vi "Am I Beside Destination.vi"(2 "Max Distance per step":cdb, 3 "Destination Location":cdb, 4 "Allowed Directions to move":T1[](array[typedef]), 5 "Current Location":cdb) -> (0 "Am I beside Destination ?":bool, 1 "Direction to Destination":T1)   [LabVIEW 2020, in "AoC 2022.lvlib"]
uses:
  AoC 2022.lvlib
  Direction.ctl
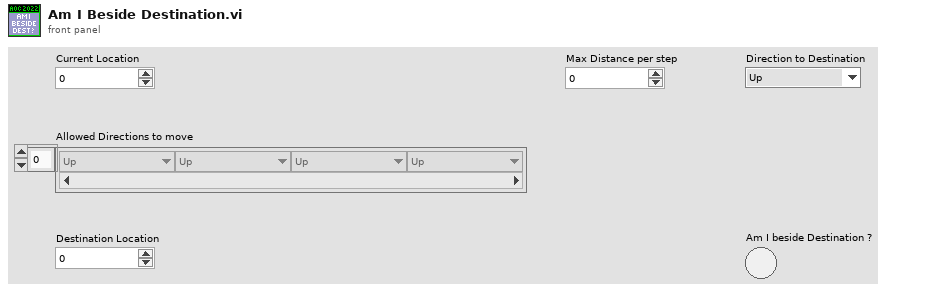
[diagram p1: front panel]
types:
  T1 = typedef "AoC 2022.lvlib/Direction.ctl" = enum16{"Up", "UpRight", "Right", "DownRight", "Down", "DownLeft", "Left", "UpLeft", "Stay"}
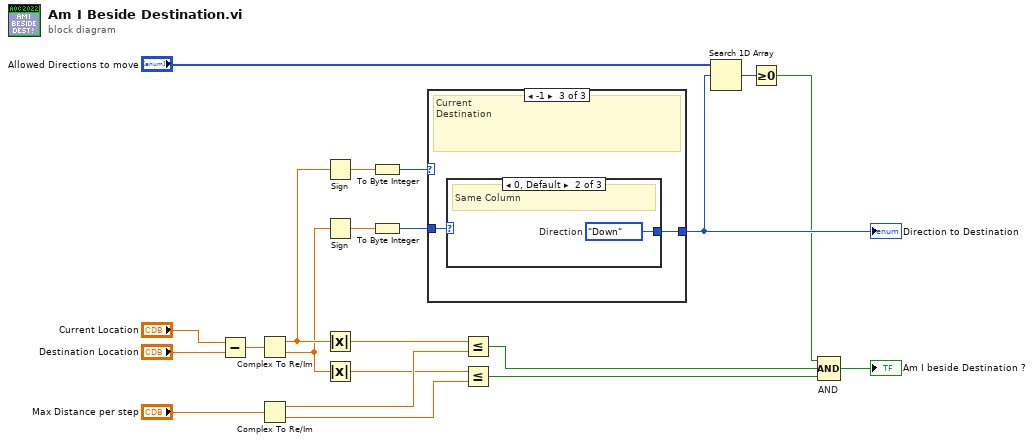
[diagram p0: block diagram]
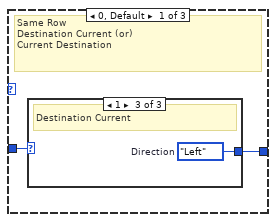
[diagram p2: hidden frame]
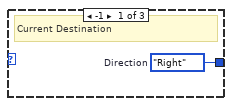
[diagram p3: hidden frame]
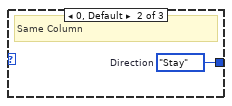
[diagram p4: hidden frame]
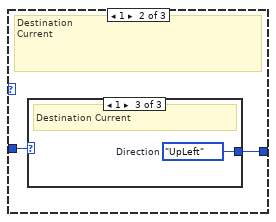
[diagram p5: hidden frame]
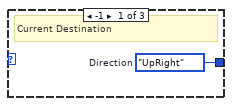
[diagram p6: hidden frame]
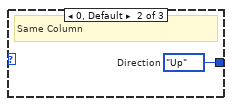
[diagram p7: hidden frame]
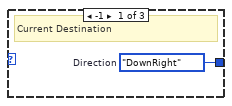
[diagram p8: hidden frame]
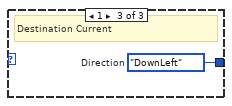
[diagram p9: hidden frame]
diagram:
  n1 = Subtract(x="Current Location", y="Destination Location") -> (x-y=w18:cdb)
  n2 = Complex To Re/Im(x + iy=w18) -> (x=w10:dbl, y=w9:dbl)
  n3 = Complex To Re/Im(x + iy="Max Distance per step") -> (x=w16:dbl, y=w15:dbl)
  n4 = Sign(1:w10) -> (0:w7:dbl)
  n5 = Sign(1:w9) -> (0:w8:dbl)
  n6 = Absolute Value(x=w10) -> (abs(x)=w19:dbl)
  n7 = Absolute Value(x=w9) -> (abs(x)=w14:dbl)
  n8 = To Byte Integer(number=w7) -> (8bit integer=w6:i8)
  n9 = To Byte Integer(number=w8) -> (8bit integer=w5:i8)
  n10 = case shown="-1" w6 {
    tunnel: w5 -> [w22 w27 w32]
    tunnel: [w23 w28 w33] -> w3
    frame 0, Default {
      # "Same Row\nDestination Current (or)\nCurrent Destination"
      n11 = case shown="1" w22 {
        tunnel: [w24 w25 w26] -> w23
        frame -1 {
          w24 = Direction."Right"  # Direction
          # "Current Destination"
        }
        frame 0, Default {
          w25 = Direction."Stay"  # Direction
          # "Same Column"
        }
        frame 1 {
          w26 = Direction."Left"  # Direction
          # "Destination Current"
        }
      }
    }
    frame 1 {
      # "Destination\nCurrent"
      n12 = case shown="1" w27 {
        tunnel: [w29 w30 w31] -> w28
        frame -1 {
          w29 = Direction."UpRight"  # Direction
          # "Current Destination"
        }
        frame 0, Default {
          w30 = Direction."Up"  # Direction
          # "Same Column"
        }
        frame 1 {
          w31 = Direction."UpLeft"  # Direction
          # "Destination Current"
        }
      }
    }
    frame -1 {
      # "Current\nDestination"
      n13 = case shown="0, Default" w32 {
        tunnel: [w34 w35 w36] -> w33
        frame -1 {
          w34 = Direction."DownRight"  # Direction
          # "Current Destination"
        }
        frame 0, Default {
          w35 = Direction."Down"  # Direction
          # "Same Column"
        }
        frame 1 {
          w36 = Direction."DownLeft"  # Direction
          # "Destination Current"
        }
      }
    }
  }
  "Direction to Destination" <- w3
  n14 = Less Or Equal?(x=w19, y=w16) -> (x <= y?=w13:bool)
  n15 = Less Or Equal?(x=w14, y=w15) -> (x <= y?=w12:bool)
  n16 = Search 1D Array(1D array="Allowed Directions to move", element=w3) -> (index of element=w2:i32)  [unwired: 1 in]
  n17 = Greater Or Equal To 0?(x=w2) -> (x >= 0?=w1:bool)
  n18 = Compound Arithmetic op=AND "AND"(w1, w13, w12) -> (→"Am I beside Destination ?":bool)
